vi "SetMsg.vi"(7 "Msg":refnum<class "Msg.lvclass">, 11 "Msg":T1 {"Metadata"."AbsoluteTime" format="%<%x %.3X>T"}) -> (5 "Msg":refnum<class "Msg.lvclass">)   [LabVIEW 2020, in "_Template.lvlib" / "{{Msg}}.lvlib" / "Msg.lvclass"]
uses:
  Msg.lvclass
  Msg.lvclass/Msg.ctl
  jettl/jettl/Lifecycle.ctl
  jettl/jettl/jettl.lvlib
  jettl/jettl/Metadata.ctl
  Msg.ctl
  {{Msg}}.lvlib
  jettl/jettl/Metadata/Metadata.lvclass
  jettl/jettl/Origin.ctl
panel:
  # "This front panel should not be manipulated."
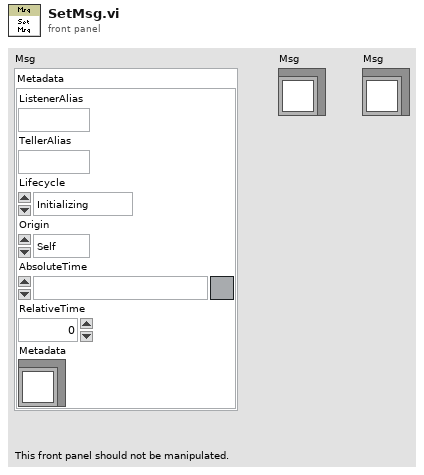
[diagram p1: front panel]
types:
  T1 = typedef "_Template.lvlib/{{Msg}}.lvlib/Msg.ctl" = cluster{"Metadata":T2}
  T2 = typedef "jettl.lvlib/Metadata.ctl" = cluster{"ListenerAlias":string, "TellerAlias":string, "Lifecycle":T3, "Origin":T4, "AbsoluteTime":timestamp, "RelativeTime":dbl, "Metadata":refnum<class "Metadata.lvclass">}
  T3 = typedef "jettl.lvlib/Lifecycle.ctl" = enum16{"Initializing", "SettingUp", "Starting", "Running", "Stopping", "TearingDown", "Terminated"}
  T4 = typedef "jettl.lvlib/Origin.ctl" = enum16{"Self", "Parent", "Child"}
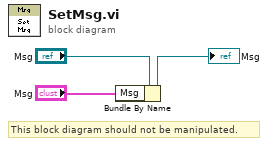
[diagram p0: block diagram]
diagram:
  # "This block diagram should not be manipulated."
  n1 = Bundle By Name(cluster="Msg", "Msg"="Msg") -> (→"Msg":refnum<class "Msg.lvclass">)
